vi "Navx get values.vi"() -> (3 "YPRH":T1)   [LabVIEW 2014]
uses:
  navx-mxp/roborio/labview/navX-MXP Library/COMMON/TypeDefs/Data TypeDefs/navX YPRH Data.ctl
  Navx data.vi
  navx-mxp/roborio/labview/navX-MXP Library/navX-MXP IMU.lvlib
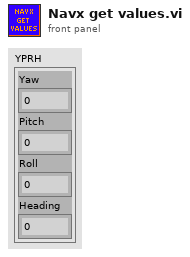
[diagram p1: front panel]
types:
  T1 = typedef "navX-MXP IMU.lvlib/navX YPRH Data.ctl" = cluster{"Yaw":dbl, "Pitch":dbl, "Roll":dbl, "Heading":dbl}
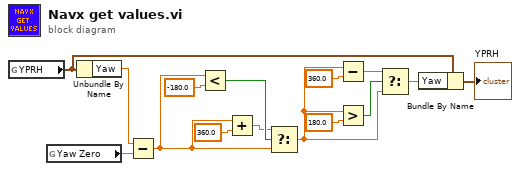
[diagram p0: block diagram]
diagram:
  n1 = global read "Navx data.vi" "YPRH"() -> (w12:T1)
  n2 = global read "Navx data.vi" "Yaw Zero"() -> (w13:dbl)
  n3 = Unbundle By Name(w12) -> ("Yaw"=w14:dbl)
  n4 = Subtract(x=w14, y=w13) -> (x-y=w7:dbl)
  n5 = Less?(x=w7, y=-180.0) -> (x < y?=w10:bool)
  n6 = Add(x=w7, y=360.0) -> (x+y=w8:dbl)
  n7 = Select(t=w8, s=w10, f=w7) -> (s? t:f=w2:dbl)
  n8 = Subtract(x=w2, y=360.0) -> (x-y=w3:dbl)
  n9 = Greater?(x=w2, y=180.0) -> (0:w5:bool)
  n10 = Select(t=w3, s=w5, f=w2) -> (s? t:f=w1:dbl)
  n11 = Bundle By Name(cluster=w12, "Yaw"=w1) -> (→"YPRH":T1)
